vi "zmq_errno.vi"(2 "retval":i32, 3 "error in":errorcluster) -> (0 "again?":bool, 1 "error out":errorcluster)   [LabVIEW 2020, in "zeromq.lvlib"]
doc: "C API calls return a value indicating success. If <b>retval</b> is negative, a description of the error is pulled from the ZMQ library.\n\nDetailed API documentation: http://api.zeromq.org/3-2:zmq-strerror"
uses:
  zeromq.lvlib
panel:
  # "ØMQ"
  # "labview"
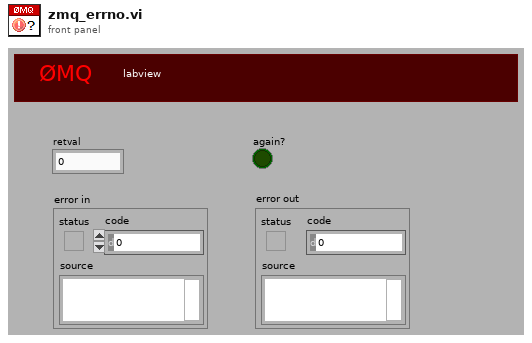
[diagram p1: front panel]
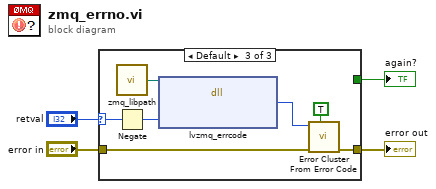
[diagram p0: block diagram]
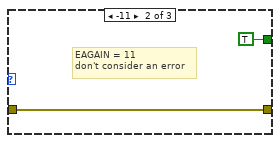
[diagram p3: hidden frame]
diagram:
  n1 = case shown="Default" "retval" {
    selector: "retval" -> [_ _ w11]
    tunnel: [w5 w7 w13] -> w2
    tunnel: "error in" -> [w5 w7 w12]
    tunnel: [_ TRUE _] -> w1
    frame 0.. {
      # "return val >= 0 is success"
    }
    frame -11 {
      # "EAGAIN = 11\ndon't consider an error"
    }
    frame Default {
      n2 = call "zmq_libpath.vi"() -> ("path"=w8:path)
      n3 = Negate(x=w11) -> (-x=w10:i32)
      n4 = dll-call lib="?" fn="lvzmq_errcode" ("zmq_labview.dll:lvzmq_strerror")(path in=w8, "retval"=w10) -> ("return type"=w9:i32)  [unwired: 3 in, 2 out]
      n5 = call "Error Cluster From Error Code.vi"("show call chain? (False)"=TRUE, "error in (no error)"=w12, "error code (0)"=w9) -> ("error out"=w13:errorcluster)  [unwired: 6 in]
    }
  }
  "error out" <- w2
  "again?" <- w1
